vi "获取所有表名.vi"(8 "error in (no error)":errorcluster, 11 "数据库连接引用 i":T1) -> (0 "error out":errorcluster, 2 "表名":string[](array[string]), 3 "数据库连接引用 o":T1)   [LabVIEW 2017]
uses:
  <vilib>/addons/database/Connection.llb/Conn ObjectReference.ctl
  <vilib>/addons/database/NI_Database_API.lvlib
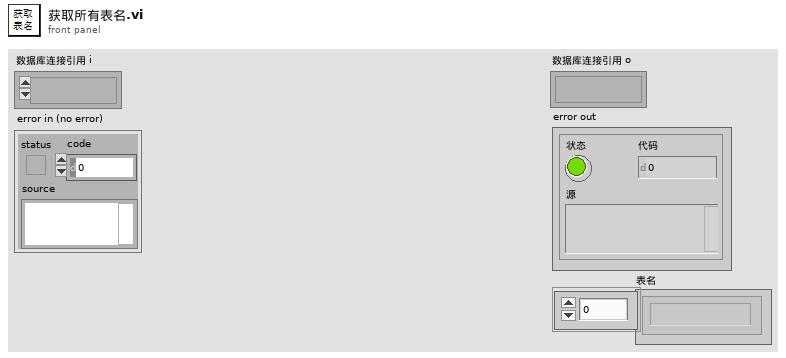
[diagram p1: front panel]
types:
  T1 = typedef "NI_Database_API.lvlib/Conn ObjectReference.ctl" = refnum<k1>
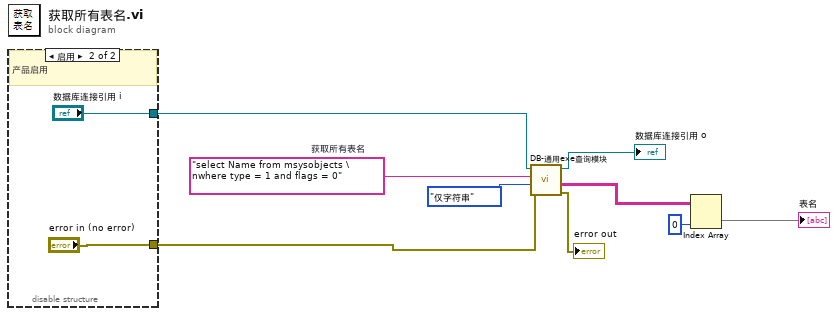
[diagram p0: block diagram]
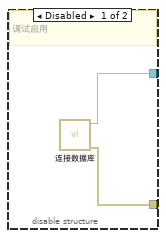
[diagram p2: hidden frame]
diagram:
  w8 = "select Name from msysobjects \nwhere type = 1 and flags = 0"  # 获取所有表名
  n1 = disable-structure shown="启用" {
    disable-tunnel: [w11 "数据库连接引用 i"] -> w2
    disable-tunnel: [w10 "error in (no error)"] -> w1
    frame Disabled {
      # "调试启用"
      n2 = call "连接数据库.vi"() -> ("error out"=w10:errorcluster, "connection reference"=w11:T1)  [unwired: 10 in]
    }
    frame Enabled {
      # "产品启用"
    }
  }
  n3 = call "DB-通用exe查询模块.vi"("error in (no error)"=w1, "解析模式"=enum16{"仅数值", "仅字符串", "数值与字符串"}."仅字符串", "SQL query"=w8, "数据库连接引用"=w2) -> ("error out"=→"error out":errorcluster, "字符串数据"=w5:string[][], "数据库连接引用out"=→"数据库连接引用 o":T1)  [unwired: 3 in, 2 out]
  n4 = Index Array(array=w5, index (col)=0 ("禁用的索引 (列)")) -> (element=→"表名":string[])  [unwired: 1 in]
